vi "Generate Event.vi"(4 "Error In":errorcluster, 6 "Response Notifier":string, 7 "Graph Name":string) -> (0 "Error Out":errorcluster)   [LabVIEW 2020, in "Read Graph Data.lvlib"]
uses:
  Read Graph Data.lvlib
  _typedefs/Event Data.ctl
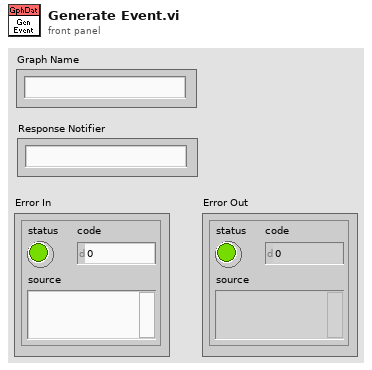
[diagram p1: front panel]
types:
  T1 = typedef "Read Graph Data.lvlib/Event Data.ctl" = cluster{"Graph Name":string, "Response Notifier":string}
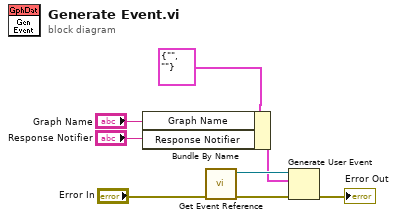
[diagram p0: block diagram]
diagram:
  n1 = Bundle By Name(cluster=T1 {"Graph Name"="", "Response Notifier"=""} ("event data"), "Graph Name"="Graph Name", "Response Notifier"="Response Notifier") -> (w3:T1)
  n2 = call "Get Event Reference.vi"("error in (no error)"="Error In") -> ("error out"=w7:errorcluster, "Read Graph Data"=w6:refnum<user-event>)  [unwired: 5 in]
  n3 = Generate User Event(user event=w6, event data cluster=w3, error in=w7) -> (error out=→"Error Out":errorcluster)  [unwired: 1 in, 1 out]
